vi "Periodic Tasks.vi"(8 "error in":errorcluster) -> ()   [LabVIEW 2023]
doc: "This VI runs in parallel to other tasks. It can contain as many user-defined periodic loops as you need. These can carry out PID or other sorts of timed response."
uses:
  <vilib>/Rock Robotics/WPI/ThirdParty/REV Robotics/REVLib/Typedef/Spark MAX Control Type.ctl
  <vilib>/Rock Robotics/WPI/Utilities/WPI_GetSetVariantRefNum.vi
panel:
  in  "Right Setpoint":dbl(slide) scale=-5700.0..5700.0
  out "Right PID Chart":T1(graph)
  in  "Right PID Constants":T2={"P Gain"=0.0, "I Gain"=0.0, "D Gain"=0.0, "F Gain"=0.0, "I Zone"=0.0, "Min Output"=-1.0, "Max Output"=1.0} {"Max Output" min=-1.0 max=1.0 step=0.01; "Min Output" min=-1.0 max=1.0 step=0.01; "I Zone" step=0.01; "F Gain" step=0.01; "D Gain" step=0.01; "I Gain" step=0.01; "P Gain" min=0.0 step=0.01}
  in  "Left Setpoint":dbl(slide) scale=-5700.0..5700.0
  out "Left PID Chart":T1(graph)
  in  "Left PID Constants":T2={"P Gain"=0.0, "I Gain"=0.0, "D Gain"=0.0, "F Gain"=0.0, "I Zone"=0.0, "Min Output"=-1.0, "Max Output"=1.0} {"Max Output" min=-1.0 max=1.0 step=0.01; "Min Output" min=-1.0 max=1.0 step=0.01; "I Zone" step=0.01; "F Gain" step=0.01; "D Gain" step=0.01; "I Gain" step=0.01; "P Gain" min=0.0 step=0.01}
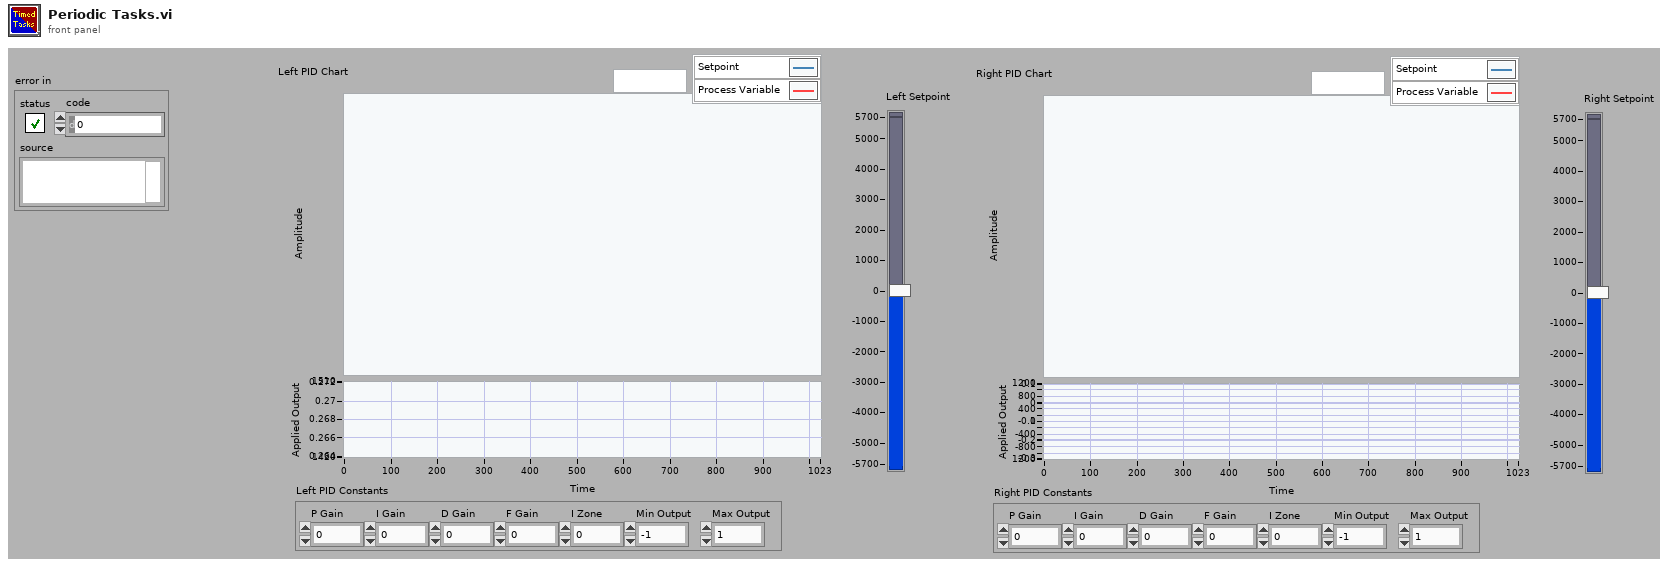
[diagram p1: front panel]
types:
  T1 = cluster{"Sensor Velocity":dbl, "Setpoint":dbl, "Applied Output":dbl}
  T2 = cluster{"P Gain":dbl, "I Gain":dbl, "D Gain":dbl, "F Gain":dbl, "I Zone":dbl, "Min Output":dbl, "Max Output":dbl}
  T3 = typedef "WPI_JoystickDevRef.ctl" = cluster{"Device":T4}
  T4 = typedef "WPI_JoystickDeviceEnum.ctl" = enum16{"USB 0", "USB 1", "USB 2", "USB 3", "USB 4", "USB 5"}
  T5 = typedef "WPI_RobotDriveDevRef.ctl" = cluster{"DevStatus":errorcluster, "Motors[]":T6[], "Square Inputs":bool, "Max Output":dbl}
  T6 = typedef "WPI_MotorControlDeviceRef.ctl" = cluster{"DeviceStatus":errorcluster, "Type":T7, "PWM":cluster{"PWM Channel":T8, "DeadBand":T9}, "CAN":cluster{"Device Number":u8, "SetOutput VI Ref":variant, "GetOutput VI Ref":variant, "Enable VI Ref":variant, "Disable VI Ref":variant, "Data":variant}, "Invert":bool, "DIO PWM":cluster{"PWM \"Enable\" Channel":T8, "DIOChannel":T10, "PWM Rate":dbl}}
  T7 = typedef "WPI_MotorControlType.ctl" = enum16{"PWM", "CAN", "DIO PWM"}
  T8 = typedef "FPGA_DIOPWMChannel.ctl" = enum8{"PWM 0", "PWM 1", "PWM 2", "PWM 3", "PWM 4", "PWM 5", "PWM 6", "PWM 7", "PWM 8", "PWM 9", "PWM MXP 0", "PWM MXP 1", "PWM MXP 2", "PWM MXP 3", "PWM MXP 4", "PWM MXP 5", "PWM MXP 6", "PWM MXP 7", "PWM MXP 8", "PWM MXP 9", "Invalid"}
  T9 = typedef "WPI_PWMDeadband.ctl" = cluster{"Name":string, "maxPositivePwm":i32, "minPositivePwm":i32, "centerPwm":i32, "maxNegativePwm":i32, "minNegativePwm":i32, "angularRange":u16}
  T10 = typedef "FPGA_DIOChannel.ctl" = enum8{"DIO 0", "DIO 1", "DIO 2", "DIO 3", "DIO 4", "DIO 5", "DIO 6", "DIO 7", "DIO 8", "DIO 9", "DIO MXP 0", "DIO MXP 1", "DIO MXP 2", "DIO MXP 3", "DIO MXP 4", "DIO MXP 5", "DIO MXP 6", "DIO MXP 7", "DIO MXP 8", "DIO MXP 9", "DIO MXP 10", "DIO MXP 11", "DIO MXP 12", "DIO MXP 13", "DIO MXP 14", "DIO MXP 15", "SPI Port CS1", "SPI Port CS2", "SPI Port CS3", "SPI Port MISO", "SPI Port MOSI", "Invalid"}
  T11 = cluster{"JoystickDevRef":T3, "RobotDriveDevRef":T5}
  T12 = typedef "Spark MAX Control Type.ctl" = enum16{"Percent VBus", "Voltage", "Velocity", "Position", "Smart Motion", "Current", "Smart Velocity"}
  T13 = cluster{"P Gain":bool, "I Gain":bool, "D Gain":bool, "F Gain":bool, "I Zone":bool, "Min Output":bool, "Max Output":bool}
  T14 = cluster{"Sensor Velocity":dbl, "Right Setpoint":dbl, "Applied Output":dbl}
  T15 = cluster{"Sensor Velocity":dbl, "Left Setpoint":dbl, "Applied Output":dbl}
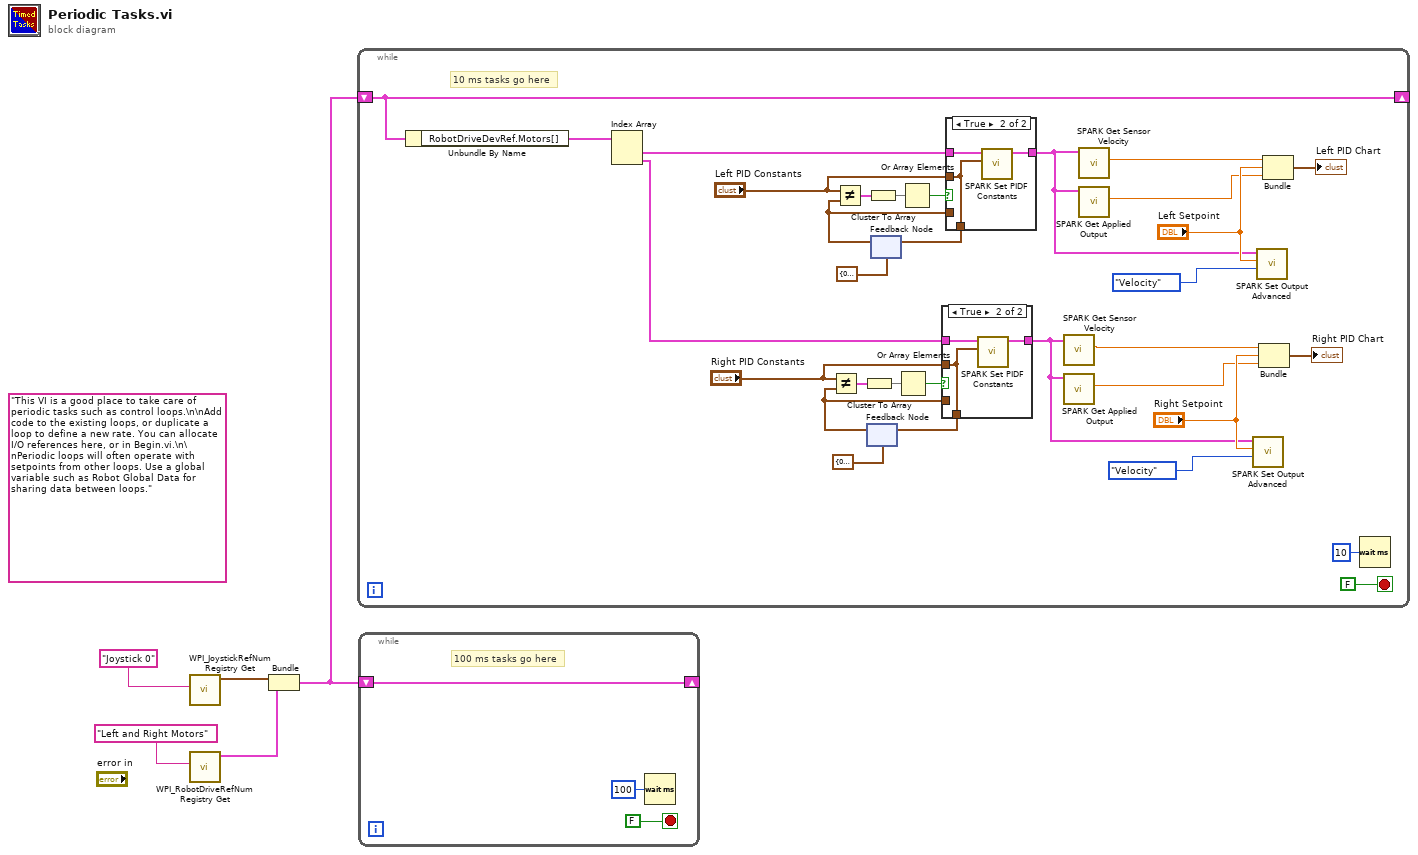
[diagram p0: block diagram]
diagram:
  (unwired) "This VI is a good place to take care of periodic tasks such as control loops.\n\nAdd code to the existing loops, or duplicate a loop to define a new rate. You can allocate I/O references here, or in Begin.vi.\n\nPeriodic loops will often operate with setpoints from other loops. Use a global variable such as Robot Global Data for sharing data between loops."
  n1 = call <vilib>:"WPI_JoystickRefNum Registry Get.vi"("refnum name"="Joystick 0") -> ("JoystickDevRef"=w3:T3)  [unwired: 1 in, 9 out]
  n2 = call <vilib>:"WPI_RobotDriveRefNum Registry Get.vi"("refnum name"="Left and Right Motors") -> ("RobotDriveDevRef"=w2:T5)  [unwired: 1 in, 9 out]
  n3 = Bundle("JoystickDevRef"=w3, "RobotDriveDevRef"=w2) -> (w1:T11)  [unwired: 1 out]
  n4 = while {
    shift-right: [w25] -> _
    shift-left: w1 -> [w25]
    stop <- FALSE stop-if-true
    # "10 ms tasks go here"
    n5 = Unbundle By Name(w25) -> ("RobotDriveDevRef.Motors[]"=w24:T6[])
    n6 = Index Array(array=w24) -> (element #1=w13:T6, element #2=w12:T6)  [unwired: 2 in]
    n7 = feedback #1(T2 {"P Gain"=0.0, "I Gain"=0.0, "D Gain"=0.0, "F Gain"=0.0, "I Zone"=0.0, "Min Output"=0.0, "Max Output"=0.0} ("PID Constants")) -> (w20:T2)
    n8 = Not Equal?(x="Right PID Constants", y=w20) -> (x != y?=w14:T13)
    n9 = Cluster To Array(cluster=w14) -> (array=w15:bool[])
    n10 = feedback #2(T2 {"P Gain"=0.0, "I Gain"=0.0, "D Gain"=0.0, "F Gain"=0.0, "I Zone"=0.0, "Min Output"=0.0, "Max Output"=0.0} ("PID Constants")) -> (w32:T2)
    n11 = Not Equal?(x="Left PID Constants", y=w32) -> (x != y?=w26:T13)
    n12 = Cluster To Array(cluster=w26) -> (array=w27:bool[])
    n13 = Or Array Elements(Boolean array=w15) -> (logical OR=w17:bool)
    n14 = Or Array Elements(Boolean array=w27) -> (logical OR=w29:bool)
    n15 = case shown="True" w17 {
      tunnel: w12 -> [w38 w42]
      tunnel: "Right PID Constants" -> [_ w40]
      tunnel: [w39 w40] -> w19
      tunnel: w20 -> [w39 _]
      tunnel: [w38 w41] -> w7
      frame False {
      }
      frame True {
        n16 = call <vilib>:"SPARK Set PIDF Constants.vi"("PID Constants"=w40, "MotorControlDeviceRef"=w42) -> ("MotorControlDeviceRef"=w41:T6)  [unwired: 8 in, 1 out]
      }
    }
    n17 = feedback-in #1(w19) -> ()
    n18 = case shown="True" w29 {
      tunnel: w13 -> [w43 w47]
      tunnel: "Left PID Constants" -> [_ w45]
      tunnel: [w44 w45] -> w31
      tunnel: w32 -> [w44 _]
      tunnel: [w43 w46] -> w10
      frame False {
      }
      frame True {
        n19 = call <vilib>:"SPARK Set PIDF Constants.vi"("PID Constants"=w45, "MotorControlDeviceRef"=w47) -> ("MotorControlDeviceRef"=w46:T6)  [unwired: 8 in, 1 out]
      }
    }
    n20 = feedback-in #2(w31) -> ()
    n21 = call <vilib>:"SPARK Get Sensor Velocity.vi"("MotorControlDevRef in"=w7) -> ("Sensor Velocity"=w8:dbl)  [unwired: 7 in, 3 out]
    n22 = call <vilib>:"SPARK Get Applied Output.vi"("MotorControlDevRef in"=w7) -> ("Applied Output"=w6:dbl)  [unwired: 7 in, 3 out]
    n23 = call <vilib>:"SPARK Get Sensor Velocity.vi"("MotorControlDevRef in"=w10) -> ("Sensor Velocity"=w11:dbl)  [unwired: 7 in, 3 out]
    n24 = call <vilib>:"SPARK Get Applied Output.vi"("MotorControlDevRef in"=w10) -> ("Applied Output"=w9:dbl)  [unwired: 7 in, 3 out]
    n25 = call <vilib>:"SPARK Set Output Advanced.vi"("Control Mode"=Spark_MAX_Control_Type."Velocity", "Setpoint"="Right Setpoint", "MotorControlDevRef"=w7) -> ()  [unwired: 7 in, 2 out]
    n26 = call <vilib>:"SPARK Set Output Advanced.vi"("Control Mode"=Spark_MAX_Control_Type."Velocity", "Setpoint"="Left Setpoint", "MotorControlDevRef"=w10) -> ()  [unwired: 7 in, 2 out]
    n27 = Bundle("Sensor Velocity"=w8, "Right Setpoint"="Right Setpoint", "Applied Output"=w6) -> (→"Right PID Chart":T14)  [unwired: 1 in]
    n28 = Bundle("Sensor Velocity"=w11, "Left Setpoint"="Left Setpoint", "Applied Output"=w9) -> (→"Left PID Chart":T15)  [unwired: 1 in]
    n29 = Wait (ms)(milliseconds to wait=u32 10) -> ()  [unwired: 1 out]
  }
  n30 = while {
    shift-right: [w48] -> _
    shift-left: w1 -> [w48]
    stop <- FALSE stop-if-true
    # "100 ms tasks go here"
    n31 = Wait (ms)(milliseconds to wait=u32 100) -> ()  [unwired: 1 out]
  }
